vi "Set MW frequency.vi"(11 "freq":dbl) -> ()   [LabVIEW 2012]
uses:
  <vilib>/express/express arith-compare/Formula/XNode/ExpressFormulaBlockNode.xnode
panel:
  in  "GPIB Address":string="19"
  in  "band (1-26.5 GHz:20)":i32(ring)=2
  in  "resolution (1 Hz:1)":i32(ring)=1 items=["0.1 Hz", "1 Hz", "10 Hz", "100 Hz", "1 KHz", "10 KHz", "100 KHz", "1 MHz", "10 MHz", "100 MHz", "1 GHz"]
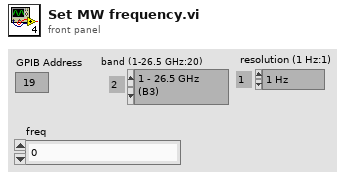
[diagram p1: front panel]
types:
  T1 = cluster{"source lock":bool, "lock frequency (Hz)":ext, "coarse tune":bool}
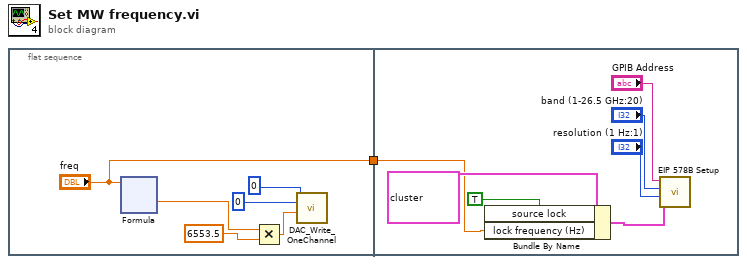
[diagram p0: block diagram]
diagram:
  n1 = flat-sequence {
    tunnel: ["freq"] -> w1
    tunnel: w1 -> [w16]
    frame #0 {
      n2 = xnode "Formula"("X1"="freq") -> ("Result"=w3:dbl)  [unwired: 1 in, 1 out]
      n3 = Multiply(x=w3, y=6553.5) -> (x*y=w6:dbl)
      n4 = call "DAC_Write_OneChannel.vi"("Value"=w6, "Channel"=u16 0, "DeviceIndex"=u64 0) -> ()  [unwired: 7 in, 2 out]
    }
    frame #1 {
      n5 = Bundle By Name(cluster=T1 {"source lock"=TRUE, "lock frequency (Hz)"=1000000000.0, "coarse tune"=TRUE} ("source locking"), "source lock"=TRUE, "lock frequency (Hz)"=w16) -> (w21:T1)
      n6 = call "EIP 578B Setup.vi"("GPIB Address"="GPIB Address", "band (1-26.5 GHz:20)"="band (1-26.5 GHz:20)", "resolution (1 Hz:1)"="resolution (1 Hz:1)", "source locking"=w21) -> ()  [unwired: 2 in, 2 out]
    }
  }
